vi "Is Connected.vi"(8 "error in (no error)":errorcluster, 11 "TCPStreamProxy in":refnum<class "TCPStream.lvclass">) -> (0 "error out":errorcluster, 2 "Connected":bool, 3 "TCPStreamProxy out":refnum<class "TCPStream.lvclass">)   [LabVIEW 2020, in "HTTP Utils.lvlib" / "TCPStream.lvclass"]
uses:
  TCPStream.lvclass
  TCPStream.lvclass/TCPStream.ctl
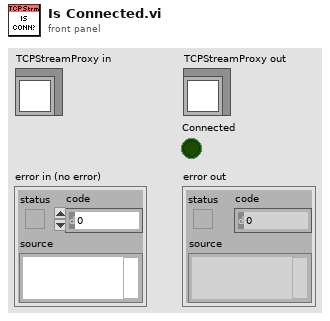
[diagram p1: front panel]
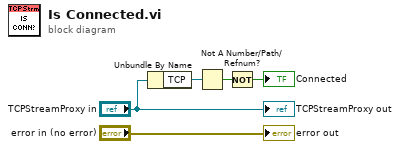
[diagram p0: block diagram]
diagram:
  n1 = Unbundle By Name("TCPStreamProxy in") -> ("TCP"=w3:refnum<k5>)
  n2 = Not A Number/Path/Refnum?(number/path/refnum=w3) -> (NaN/Path/Refnum?=w2:bool)
  n3 = Not(x=w2) -> (.not. x?=→"Connected":bool)
  "error out" <- "error in (no error)"
  "TCPStreamProxy out" <- "TCPStreamProxy in"
